vi "getParAndArgChkRes.vi"(6 "sec":string, 8 "error in":errorcluster, 9 "func":string, 10 "arg":string, 11 "Tree Refnum in":refnum<vi>) -> (0 "error out":errorcluster, 1 "Check result":string="√", 2 "par":string, 3 "Tree Refnum out":refnum<vi>)   [LabVIEW 2010]
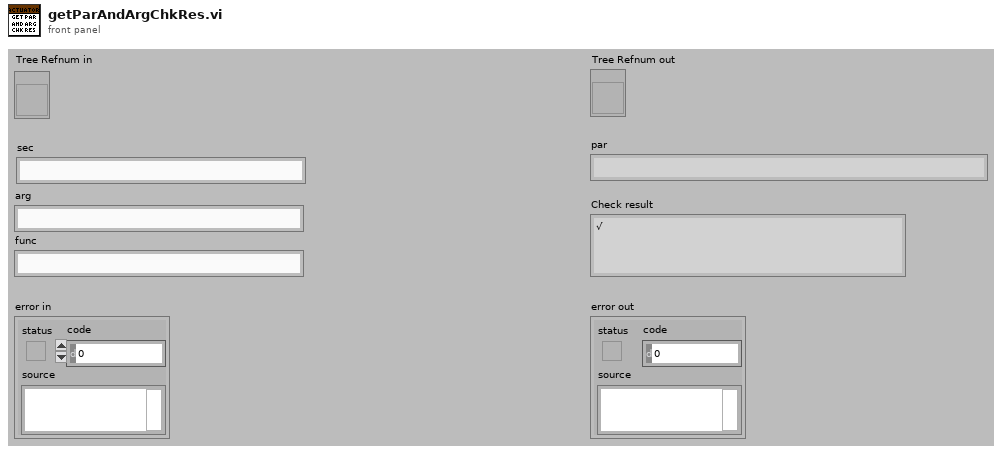
[diagram p1: front panel]
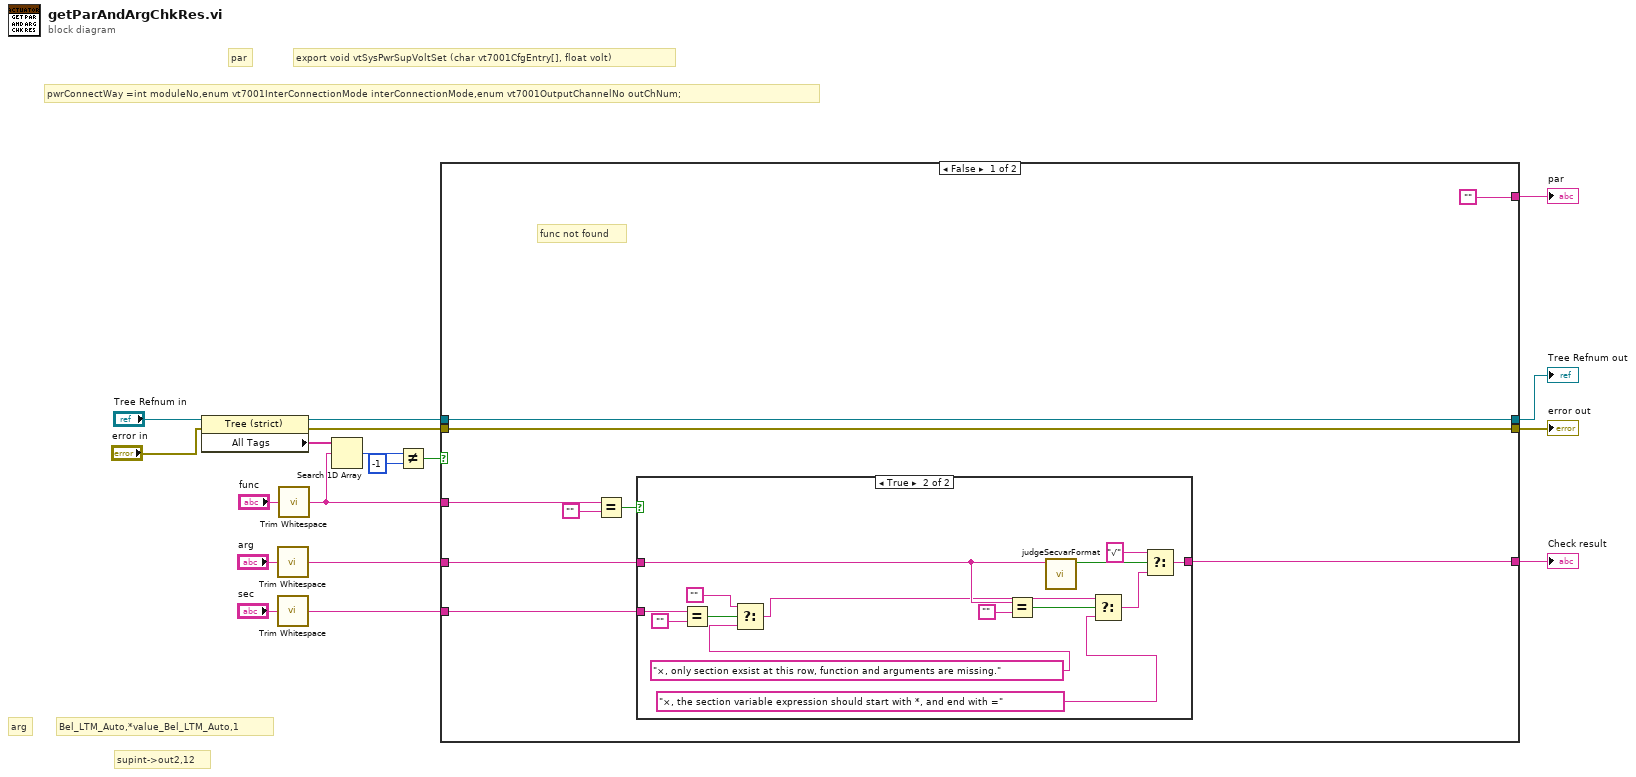
[diagram p0: block diagram]
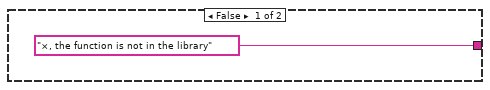
[diagram p2: hidden frame]
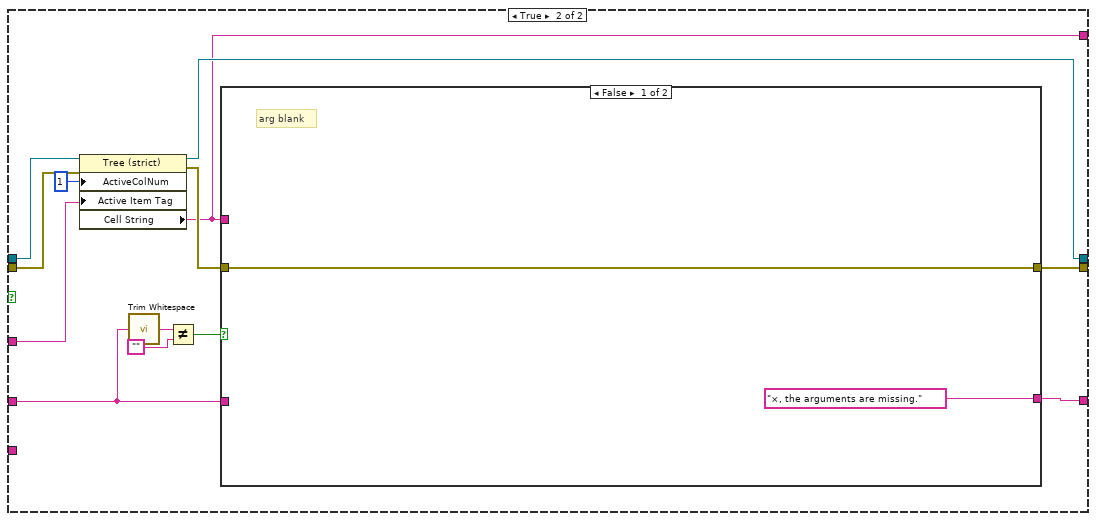
[diagram p3: hidden frame]
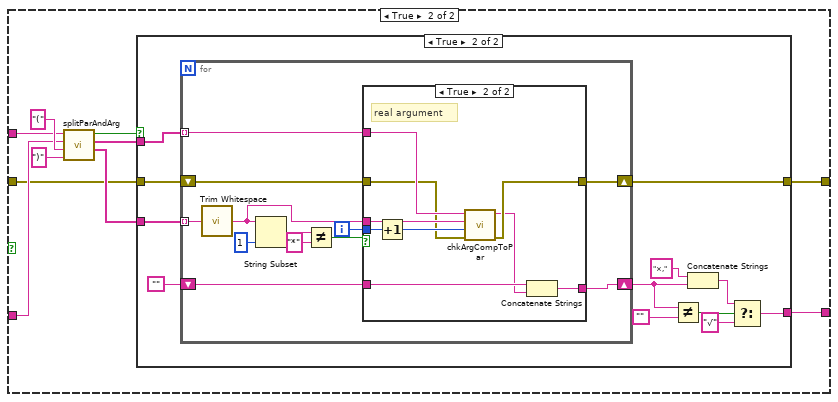
[diagram p4: hidden frame]
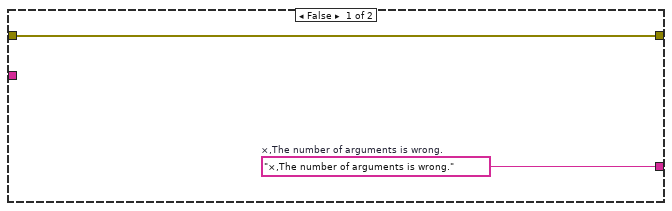
[diagram p5: hidden frame]
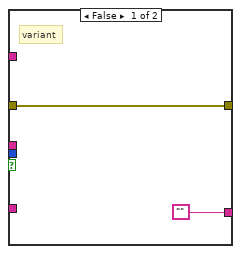
[diagram p6: hidden frame]
diagram:
  # "pwrConnectWay =int moduleNo,enum vt7001InterConnectionMode interConnectionMode,enum vt7001OutputChannelNo outChNum;"
  # "arg"
  # "par"
  # "Bel_LTM_Auto,*value_Bel_LTM_Auto,1"
  # "supint->out2,12"
  # "export void vtSysPwrSupVoltSet (char vt7001CfgEntry[], float volt)"
  n1 = property on="Property Node" class="Tree (strict)"(reference="Tree Refnum in", error in="error in") -> (reference out=w11:refnum<vi>, error out=w12:errorcluster, "All Tags"=w15:string[])
  n2 = call <vilib>:"Trim Whitespace.vi"("string"="arg") -> ("trimmed string"=w7:string)  [unwired: 1 in]
  n3 = call <vilib>:"Trim Whitespace.vi"("string"="sec") -> ("trimmed string"=w1:string)  [unwired: 1 in]
  n4 = call <vilib>:"Trim Whitespace.vi"("string"="func") -> ("trimmed string"=w8:string)  [unwired: 1 in]
  n5 = Search 1D Array(1D array=w15, element=w8) -> (index of element=w14:i32)  [unwired: 1 in]
  n6 = Not Equal?(x=w14, y=-1) -> (x != y?=w18:bool)
  n7 = case shown="False" w18 {
    tunnel: w7 -> [w24 w50]
    tunnel: w12 -> [w21 w48]
    tunnel: [w23 w55] -> w17
    tunnel: [w21 w54] -> w16
    tunnel: w11 -> [w22 w46]
    tunnel: [w22 w44] -> w10
    tunnel: w8 -> [w27 w47]
    tunnel: ["" w43] -> w3
    tunnel: w1 -> [w19 _]
    frame False {
      # "func not found"
      n8 = Equal?(x=w27, y="") -> (x = y?=w25:bool)
      n9 = case shown="True" w25 {
        tunnel: w24 -> [_ w36]
        tunnel: ["×, the function is not in the library" w41] -> w23
        tunnel: w19 -> [_ w34]
        frame False {
        }
        frame True {
          n10 = Equal?(x=w34, y="") -> (x = y?=w32:bool)
          n11 = Select(t="", s=w32, f="×, only section exsist at this row, function and arguments are missing." ("Value")) -> (s? t:f=w29:string)
          n12 = Equal?(x=w36, y="") -> (x = y?=w40:bool)
          n13 = call "judgeSecvarFormat.vi"("section variable"=w36) -> ("correct format?"=w37:bool)  [unwired: 10 in]
          n14 = Select(t=w29, s=w40, f="×, the section variable expression should start with *, and end with =" ("Value")) -> (s? t:f=w35:string)
          n15 = Select(t="√", s=w37, f=w35) -> (s? t:f=w41:string)
        }
      }
    }
    frame True {
      n16 = property class="Tree (strict)"(reference=w46, error in=w48, "ActiveColNum"=1 ("Active Cell:Active Column Number"), "Active Item Tag"=w47) -> (reference out=w44:refnum<vi>, error out=w45:errorcluster, "Cell String"=w43:string)
      n17 = call <vilib>:"Trim Whitespace.vi"("string"=w50) -> ("trimmed string"=w53:string)  [unwired: 1 in]
      n18 = Not Equal?(x=w53, y="") -> (x != y?=w51:bool)
      n19 = case shown="False" w51 {
        tunnel: w43 -> [_ w63]
        tunnel: w50 -> [_ w62]
        tunnel: w45 -> [w57 w58]
        tunnel: ["×, the arguments are missing." w67] -> w55
        tunnel: [w57 w66] -> w54
        frame False {
          # "arg blank"
        }
        frame True {
          n20 = call "splitParAndArg.vi"("paraEndMark"=")" ("regular expression"), "paraStartMark"="(" ("regular expression"), "allArguments"=w62, "allParameters"=w63) -> ("argArray"=w60:string[], "paraArray"=w61:string[], "sameNum?"=w59:bool)  [unwired: 5 in]
          n21 = case shown="True" w59 {
            tunnel: w61 -> [_ w81]
            tunnel: w60 -> [_ w80]
            tunnel: [w69 w75] -> w67
            tunnel: w58 -> [w68 w74]
            tunnel: [w68 w73] -> w66
            frame False {
              w69 = "×,The number of arguments is wrong."  # ×,The number of arguments is wrong.
            }
            frame True {
              n22 = for {
                tunnel: w81 -> [w93] mode=indexing
                tunnel: w80 -> [w83] mode=indexing
                shift-right: [w91] -> w71
                shift-left: "" -> [w92]
                shift-right: [w89] -> w73
                shift-left: w74 -> [w90]
                i -> [w84]
                n23 = call <vilib>:"Trim Whitespace.vi"("string"=w83) -> ("trimmed string"=w82:string)  [unwired: 1 in]
                n24 = String Subset(string=w82, length (rest)=1 ("length (rest)")) -> (substring=w87:string)  [unwired: 1 in]
                n25 = Not Equal?(x=w87, y="*") -> (x != y?=w85:bool)
                n26 = case shown="True" w85 {
                  tunnel: w93 -> [_ w101]
                  tunnel: w92 -> [_ w104]
                  tunnel: ["" w103] -> w91
                  tunnel: w90 -> [w94 w98]
                  tunnel: [w94 w97] -> w89
                  tunnel: w84 -> [_ w100]
                  tunnel: w82 -> [_ w102]
                  frame False {
                    # "variant"
                  }
                  frame True {
                    # "real argument"
                    n27 = Increment(x=w100) -> (x+1=w99:i32)
                    n28 = call "chkArgCompToPar.vi"("error in"=w98, "argSN"=w99, "arg"=w102, "par"=w101) -> ("error out"=w97:errorcluster, "judgement"=w96:string)  [unwired: 6 in]
                    n29 = Concatenate Strings(w104, w96) -> (w103:string)
                  }
                }
              }
              n30 = Not Equal?(x=w71, y="") -> (x != y?=w77:bool)
              n31 = Concatenate Strings("×,", w71) -> (w70:string)
              n32 = Select(t=w70, s=w77, f="√") -> (s? t:f=w75:string)
            }
          }
        }
      }
    }
  }
  "Check result" <- w17
  "error out" <- w16
  "Tree Refnum out" <- w10
  "par" <- w3
